vi "TemperatureConversion.vi"() -> ()   [LabVIEW 2017, in "Examples.lvlib"]
uses:
  Examples.lvlib
panel:
  in  "Boolean":bool
  in  "stop":bool
  out "Thermometer (C)":dbl(slide) scale=0.0..100.0
  in  "Temperature (F)":dbl(slide) scale=0.0..200.0
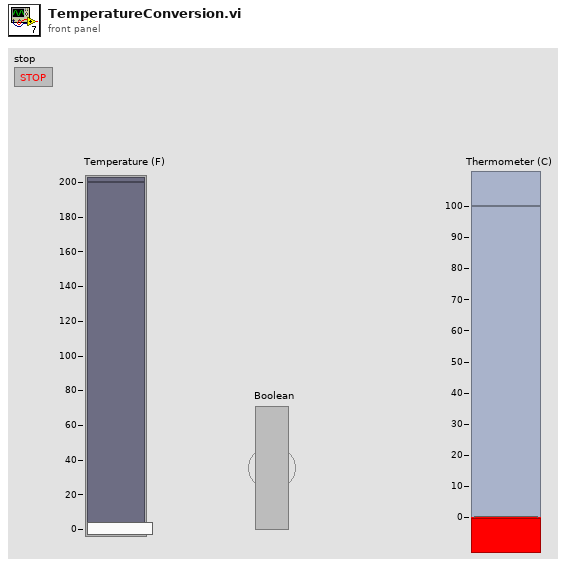
[diagram p1: front panel]
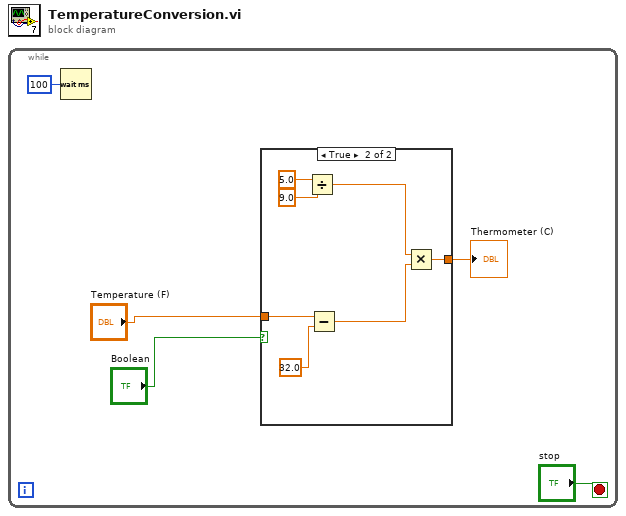
[diagram p0: block diagram]
diagram:
  n1 = while {
    stop <- "stop" stop-if-true
    n2 = Wait (ms)(milliseconds to wait=u32 100) -> ()  [unwired: 1 out]
    n3 = case shown="True" "Boolean" {
      tunnel: [w6 w8] -> w4
      tunnel: "Temperature (F)" -> [w6 w7]
      frame False {
      }
      frame True {
        n4 = Divide(x=5.0, y=9.0) -> (x/y=w10:dbl)
        n5 = Subtract(x=w7, y=32.0) -> (x-y=w9:dbl)
        n6 = Multiply(x=w10, y=w9) -> (x*y=w8:dbl)
      }
    }
    "Thermometer (C)" <- w4
  }
